vi "runScript.vi"(8 "error in (no error)":errorcluster, 9 "script":string, 10 "matlabScript":string, 11 "MatlabScripts in":refnum<class "MatlabScripts.lvclass">) -> (0 "error out":errorcluster, 3 "MatlabScripts out":refnum<class "MatlabScripts.lvclass">)   [LabVIEW 2009, in "Views.lvlib" / "ExperimentControl.lvlib" / "MatlabScripts.lvclass"]
uses:
  MatlabScripts.lvclass
  Tools/Filing/FileSystem/FileSystem.lvclass
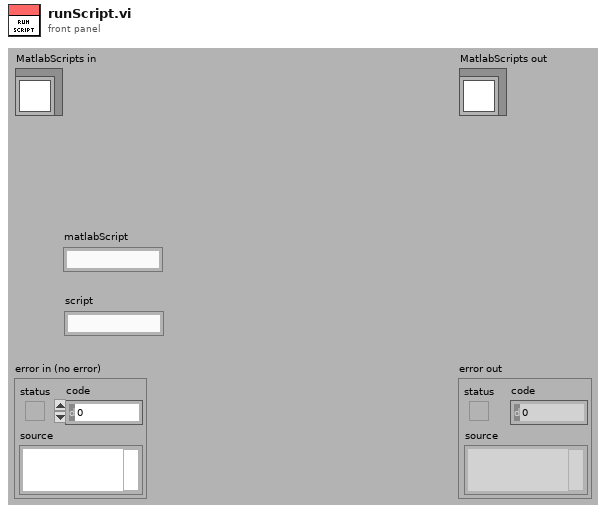
[diagram p1: front panel]
types:
  T1 = enum32{"Invalid", "Standard", "Closed", "Hidden", "Minimized", "Maximized"}
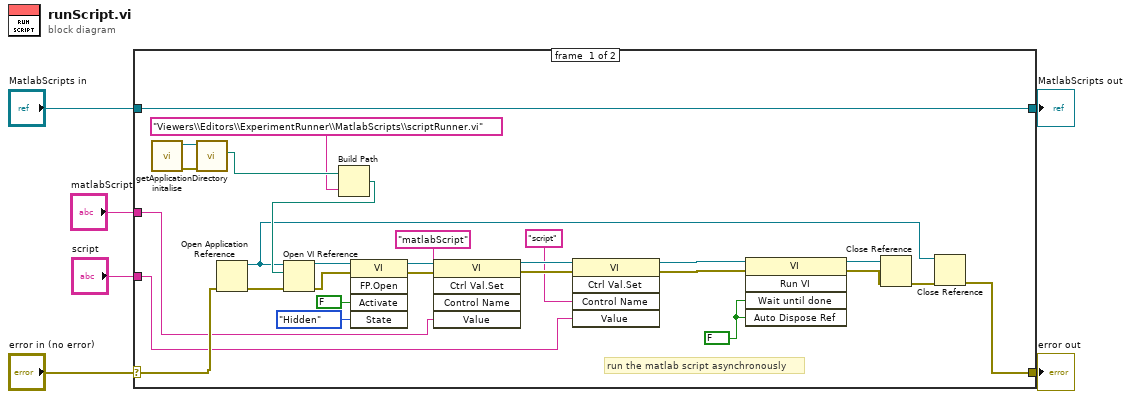
[diagram p0: block diagram]
diagram:
  n1 = case shown="No Error" "error in (no error)" {
    selector: "error in (no error)" -> [w29 w36]
    tunnel: [w12 w36] -> w5
    tunnel: [w34 w35] -> w3
    tunnel: "MatlabScripts in" -> [w34 w35]
    tunnel: "matlabScript" -> [w19 _]
    tunnel: "script" -> [w8 _]
    frame #0 {
      w17 = FALSE
      # "run the matlab script asynchronously"
      n2 = call "initalise.vi"() -> ("error out"=w32:errorcluster, "FileSystem out"=w33:refnum<class "FileSystem.lvclass">)  [unwired: 10 in]
      n3 = call-dynamic "getApplicationDirectory.vi"("error in (no error)"=w32, "FileSystem.lvclass in"=w33) -> ("ApplicationDirectory"=w31:path)  [unwired: 7 in, 2 out]
      n4 = Open Application Reference(8:w29) -> (0:w28:errorcluster, 3:w13:refnum<vi>)  [unwired: 3 in]
      n5 = Build Path(base path=w31, name or relative path="Viewers\\Editors\\ExperimentRunner\\MatlabScripts\\scriptRunner.vi") -> (appended path=w27:path)
      n6 = Open VI Reference(application reference (local)=w13, vi path=w27, error in (no error)=w28) -> (vi reference=w25:refnum<vi>, error out=w26:errorcluster)  [unwired: 3 in]
      n7 = invoke class="VI" method="FP.Open"(reference=w25, error in=w26, "Activate"=FALSE ("Activate?"), "State"=T1."Hidden") -> (reference out=w22:refnum<vi>, error out=w21:errorcluster)  [unwired: 1 in, 3 out]
      n8 = invoke class="VI" method="Ctrl Val.Set"(reference=w22, error in=w21, "Control Name"="matlabScript", "Value"=w19) -> (reference out=w18:refnum<vi>, error out=w10:errorcluster)  [unwired: 1 in, 3 out]
      n9 = invoke class="VI" method="Ctrl Val.Set"(reference=w18, error in=w10, "Control Name"="script", "Value"=w8) -> (reference out=w11:refnum<vi>, error out=w9:errorcluster)  [unwired: 1 in, 3 out]
      n10 = invoke class="VI" method="Run VI"(reference=w11, error in=w9, "Wait until done"=w17, "Auto Dispose Ref"=w17) -> (reference out=w16:refnum<vi>, error out=w15:errorcluster)  [unwired: 1 in, 3 out]
      n11 = Close Reference(reference=w16, error in (no error)=w15) -> (error out=w14:errorcluster)
      n12 = Close Reference(reference=w13, error in (no error)=w14) -> (error out=w12:errorcluster)
    }
    frame #1 {
    }
  }
  "error out" <- w5
  "MatlabScripts out" <- w3
